vi "Main Globals.vi"() -> ()   [LabVIEW 2018]
panel:
  in  "Python Version":string
  in  "Python Folder":path
  in  "Protocol Folder":path
  in  "Reports":path
  in  "Pump Position":u32=1000
  in  "Cancel":bool
  in  "Stop Script":bool
  in  "Logs Folder":path
  in  "Config Folder":path
  in  "Scripts Folder":path
  in  "Data Folder":path
  in  "Record Data":bool
  in  "Number of Samples":i16=100
  in  "Sampling Rate":i16=1000
  in  "data file path":path
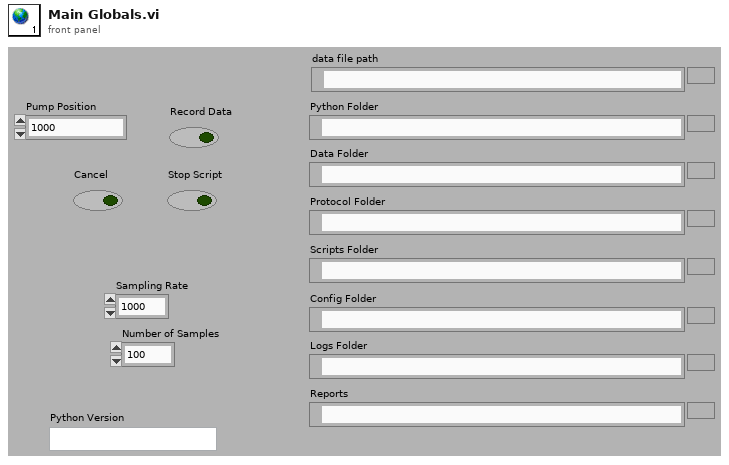
[diagram p1: front panel]
diagram:
